vi "GetLocalInstanceName.vi"(8 "error in (no error)":errorcluster, 11 "result string in":string) -> (0 "error out":errorcluster, 3 "result string out":string)   [LabVIEW 2017]
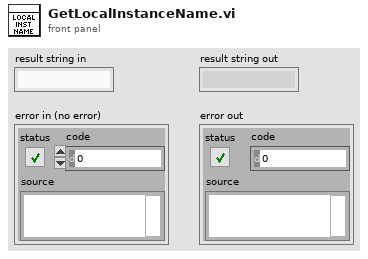
[diagram p1: front panel]
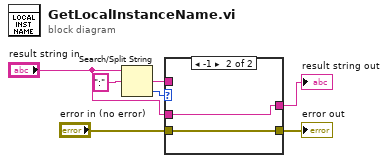
[diagram p0: block diagram]
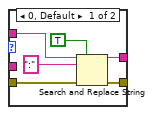
[diagram p2: hidden frame]
diagram:
  n1 = Search/Split String(string="result string in", search string/char (-)=":" ("replace string (\"\")")) -> (match + rest of string=w2:string, offset of match=w6:i32)  [unwired: 1 in, 1 out]
  n2 = case shown="-1" w6 {
    tunnel: w2 -> [w13 _]
    tunnel: "error in (no error)" -> [w11 w15]
    tunnel: [w10 w15] -> w4
    tunnel: [w9 w14] -> w5
    tunnel: "result string in" -> [_ w14]
    frame 0, Default {
      n3 = Search and Replace String(replace all?=TRUE ("replace all? (F)"), input string=w13, search string=":", error in=w11) -> (result string=w9:string, error out=w10:errorcluster)  [unwired: 4 in, 2 out]
    }
    frame -1 {
    }
  }
  "result string out" <- w5
  "error out" <- w4
